vi "THzTimeScan_830.vi"(0 "input":T1) -> (1 "loop stop":bool, 2 "x-axis":sgl[](array[numeric]), 3 "y-axis":dbl[](array[numeric]))   [LabVIEW 2010]
panel:
  out "Array":dbl[](array[numeric])
  out "String":string
  out "Read position":bool
  out "Ask position":bool
  out "Move delay":bool
  out "Read830":bool
  out "Command":string
  out "THz Signal Graph":dbl(graph)
  in  "loop stop":bool
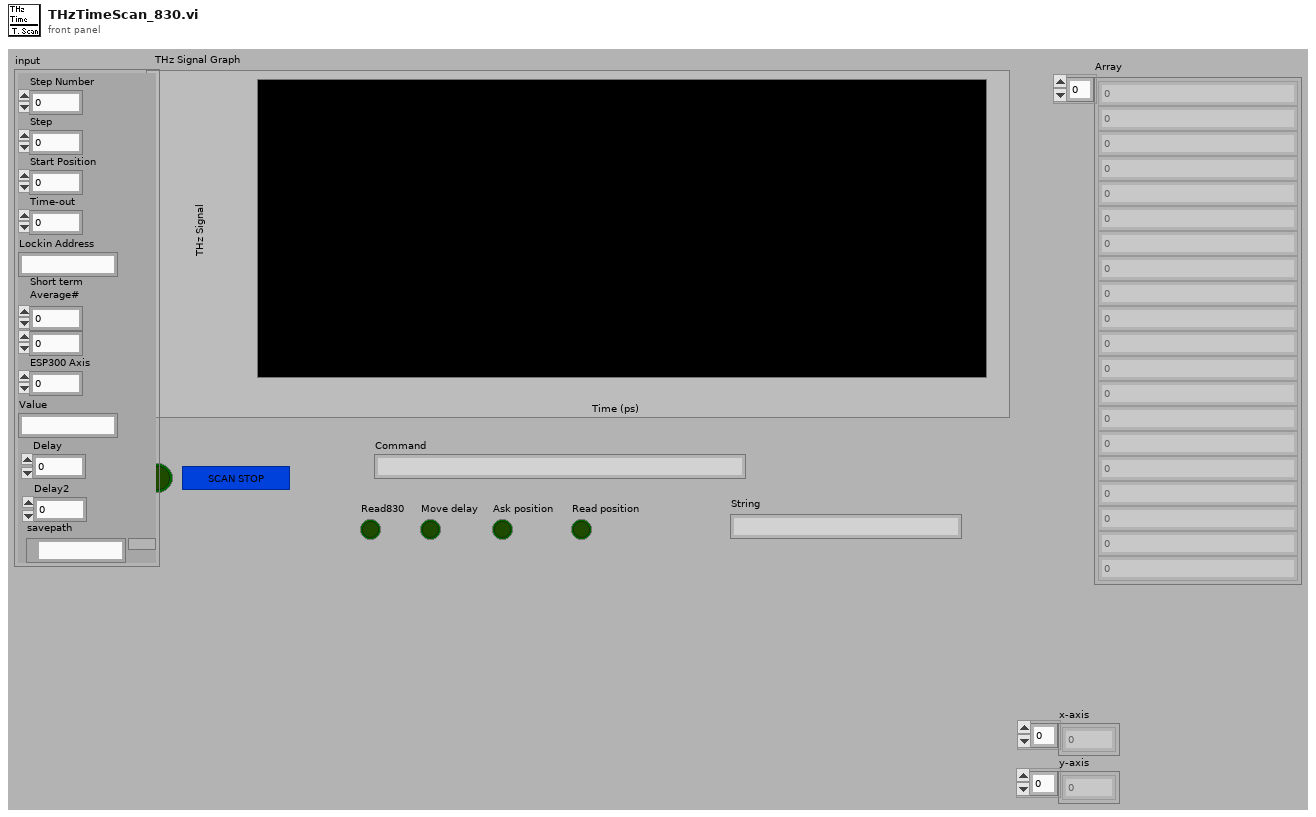
[diagram p1: front panel]
types:
  T1 = cluster{"Step Number":i32, "Step":sgl, "Start Position":sgl, "Time-out":i32, "Lockin Address":string, "Short term \nAverage#":i8, i32, "ESP300 Axis":i8, "Value":string, "Delay":dbl, "Delay2":dbl, "savepath":path}
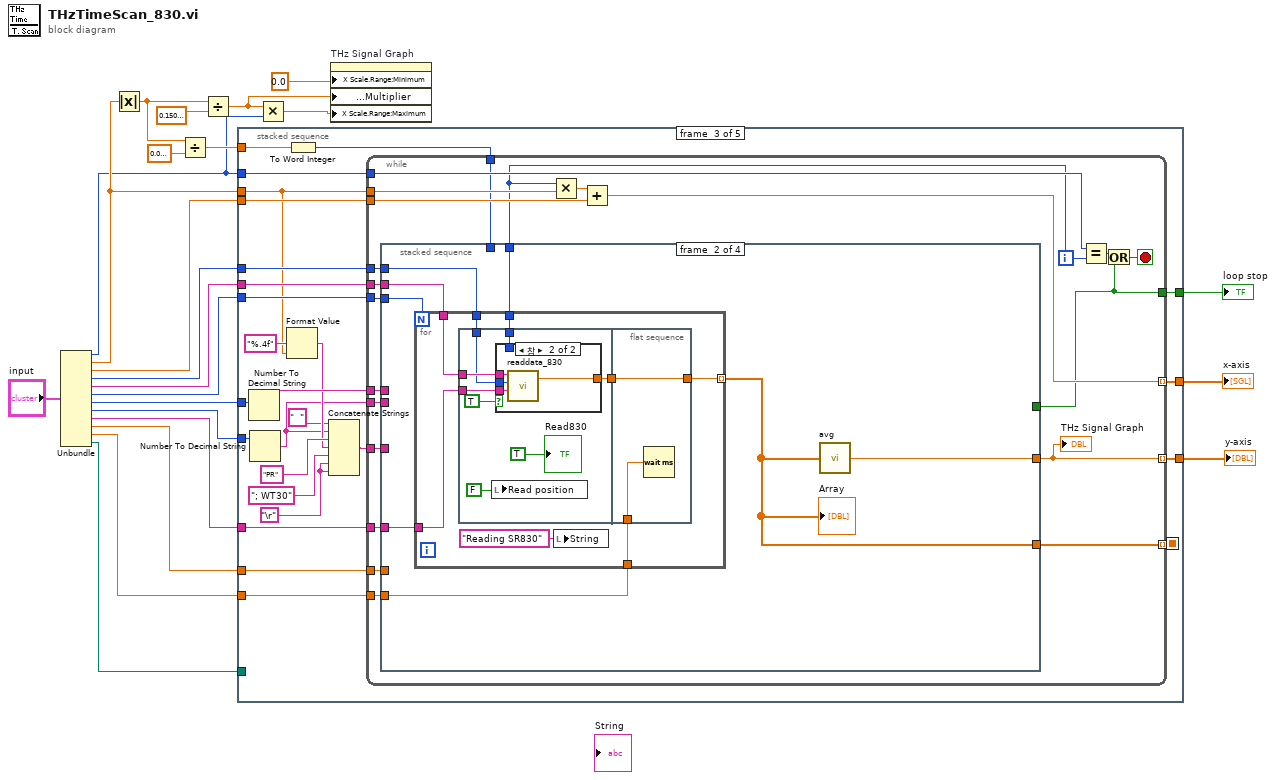
[diagram p0: block diagram]
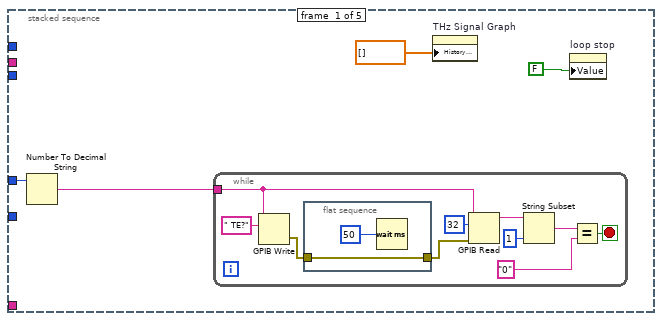
[diagram p2: hidden frame]
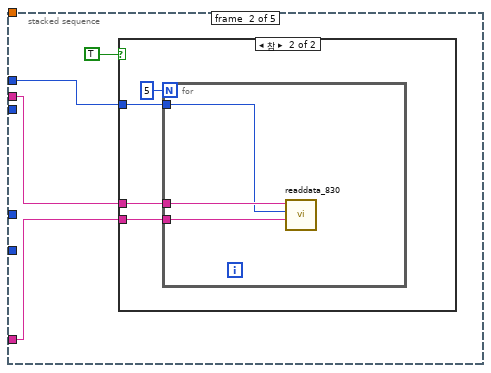
[diagram p3: hidden frame]
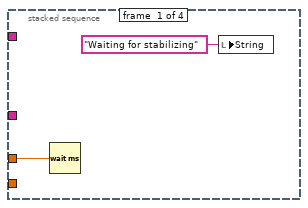
[diagram p5: hidden frame]
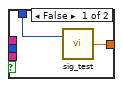
[diagram p6: hidden frame]
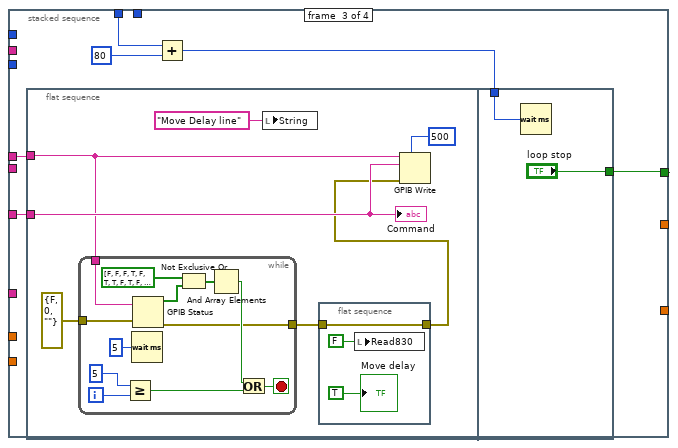
[diagram p7: hidden frame]
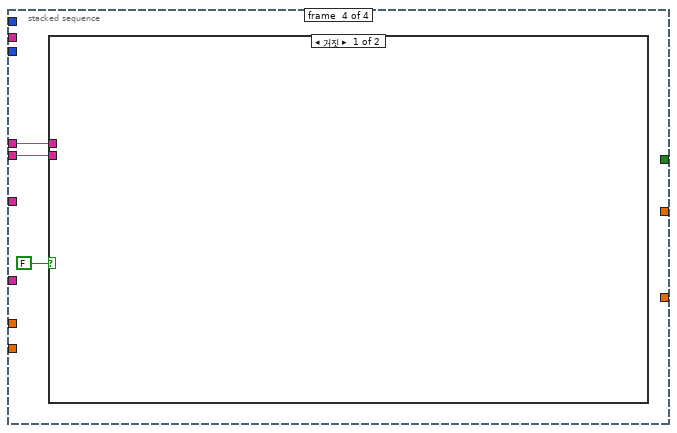
[diagram p8: hidden frame]
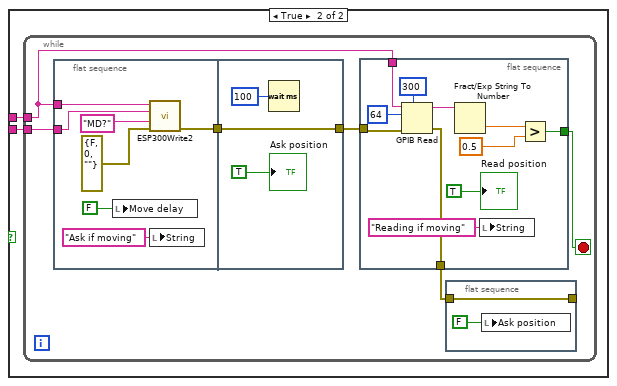
[diagram p9: hidden frame]
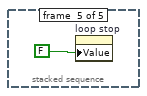
[diagram p11: hidden frame]
diagram:
  n1 = Unbundle("input") -> ("Step Number"=w8:i32, "Step"=w15:sgl, "Start Position"=w14:sgl, "Time-out"=w13:i32, "Lockin Address"=w12:string, "Short term \nAverage#"=w4:i8, w11:i32, "ESP300 Axis"=w10:i8, "Value"=w9:string, "Delay"=w3:dbl, "Delay2"=w2:dbl, "savepath"=w1:path)
  n2 = Absolute Value(x=w15) -> (abs(x)=w19:sgl)
  n3 = Divide(x=w19, y=sgl 0.004) -> (x/y=w17:sgl)
  n4 = Divide(x=w19, y=sgl 0.15) -> (x/y=w6:sgl)
  n5 = stacked-sequence {
    seq-local: [_ _ w52 _ _] -> [_ _ _ _ _]
    tunnel: w14 -> [_ _ w76 _ _]
    tunnel: w13 -> [_ w43 w75 _ _]
    tunnel: w12 -> [_ w42 w74 _ _]
    tunnel: w4 -> [_ _ w73 _ _]
    tunnel: w11 -> [w25 _ w68 _ _]
    tunnel: w10 -> [_ _ w66 _ _]
    tunnel: w9 -> [_ w41 w58 _ _]
    tunnel: [_ _ w72 _ _] -> w23
    tunnel: [_ _ w71 _ _] -> w22
    tunnel: [_ _ w70 _ _] -> w21
    tunnel: w15 -> [_ _ w64 _ _]
    tunnel: w8 -> [_ _ w69 _ _]
    tunnel: w17 -> [_ _ w63 _ _]
    tunnel: w3 -> [_ _ w54 _ _]
    tunnel: w2 -> [_ _ w53 _ _]
    tunnel: w1 -> [_ _ _ _ _]
    frame #0 {
      n6 = Number To Decimal String(number=w25) -> (decimal integer string=w24:string)  [unwired: 1 in]
      n7 = while {
        tunnel: w24 -> [w30]
        stop <- w35 stop-if-true
        n8 = GPIB Write(0:w30, 1:" TE?" ("data")) -> (6:w29:errorcluster)  [unwired: 3 in, 1 out]
        n9 = flat-sequence {
          tunnel: w29 -> [w39]
          tunnel: [w39] -> w28
          frame #0 {
            n10 = Wait (ms)(milliseconds to wait=u32 50) -> ()  [unwired: 1 out]
          }
        }
        n11 = GPIB Read(0:w30, 1:32 ("byte count"), 3:w28) -> (5:w34:string)  [unwired: 2 in, 2 out]
        n12 = String Subset(string=w34, length (rest)=1 ("offset (0)")) -> (substring=w32:string)  [unwired: 1 in]
        n13 = Equal?(x=w32, y="0") -> (x = y?=w35:bool)
      }
      n14 = property on="THz Signal Graph" class="WFChart (엄격한)"("History Data"=dbl[] []) -> ()  [unwired: 2 in, 2 out]
      n15 = property on="loop stop" class="Bool (엄격한)"("Value"=FALSE) -> ()  [unwired: 2 in, 2 out]
    }
    frame #1 {
      n16 = case shown="참" TRUE {
        tunnel: w43 -> [_ w46]
        tunnel: w42 -> [_ w45]
        tunnel: w41 -> [_ w44]
        frame False {
        }
        frame True {
          n17 = for {
            N: 5 -> [_]
            tunnel: w45 -> [w50]
            tunnel: w44 -> [w49]
            tunnel: w46 -> [w48]
            n18 = call "readdata_830.vi"("Command"=w49, "timeout"=w48, "Lockin Address"=w50) -> ()  [unwired: 1 in, 2 out]
          }
        }
      }
    }
    frame #2 {
      w57 = "\r"
      n19 = Number To Decimal String(number=w68) -> (decimal integer string=w67:string)  [unwired: 1 in]
      n20 = Number To Decimal String(number=w66) -> (decimal integer string=w55:string)  [unwired: 1 in]
      n21 = Format Value(format string="%.4f", value (0)=w64) -> (output string=w60:string)  [unwired: 1 in]
      n22 = To Word Integer(number=w63) -> (16bit integer=w62:i16)
      n23 = Concatenate Strings("  " ("string"), w55, "PR" ("Substring"), w60, "; WT30" ("string"), w57, w57) -> (w51:string)
      n24 = while {
        tunnel: [w82] -> w72
        tunnel: [w88] -> w70 mode=indexing
        tunnel: [w94] -> w71 mode=indexing
        tunnel: w69 -> [w93]
        tunnel: w64 -> [w92]
        tunnel: w76 -> [w91]
        tunnel: w75 -> [w83]
        tunnel: w74 -> [w90]
        tunnel: w73 -> [w89]
        tunnel: w67 -> [w87]
        tunnel: w51 -> [w86]
        tunnel: w62 -> [w85]
        tunnel: w58 -> [w84]
        tunnel: w55 -> [w81]
        tunnel: w54 -> [w80]
        tunnel: w53 -> [w79]
        tunnel: [w78] -> w52 mode=indexing
        i -> [w77]
        stop <- w97 stop-if-true
        n25 = stacked-sequence {
          tunnel: w90 -> [_ w104 _ _]
          tunnel: [_ w106 _ _] -> w88
          tunnel: w89 -> [_ w107 _ _]
          tunnel: w87 -> [_ _ w136 w164]
          tunnel: w86 -> [_ _ w137 _]
          tunnel: w85 -> [_ _ w135 _]
          tunnel: w84 -> [_ w105 _ _]
          tunnel: w83 -> [_ w103 _ _]
          tunnel: [_ _ w132 _] -> w82
          tunnel: w81 -> [_ _ _ w163]
          tunnel: w80 -> [w99 _ _ _]
          tunnel: w79 -> [_ w102 _ _]
          tunnel: [_ w101 _ _] -> w78
          tunnel: w77 -> [_ w100 _ _]
          frame #0 {
            n26 = Wait (ms)(milliseconds to wait=w99) -> ()  [unwired: 1 out]
            n27 = local write "String"("Waiting for stabilizing" ("String")) -> ()
          }
          frame #1 {
            n28 = for {
              N: w107 -> [_]
              tunnel: w104 -> [w112]
              tunnel: w103 -> [w115]
              tunnel: [w114] -> w101 mode=indexing
              tunnel: w105 -> [w113]
              tunnel: w102 -> [w109]
              tunnel: w100 -> [w108]
              n29 = flat-sequence {
                tunnel: w115 -> [w119]
                tunnel: w113 -> [w120]
                tunnel: w112 -> [w121]
                tunnel: [w118] -> w110
                tunnel: w108 -> [w116]
                tunnel: [w131] -> w114
                tunnel: w110 -> [w131]
                tunnel: w109 -> [w130]
                frame #0 {
                  n30 = local write "Read position"(FALSE ("Read position")) -> ()
                  n31 = case shown="참" TRUE {
                    tunnel: w121 -> [_ w129]
                    tunnel: w120 -> [_ w128]
                    tunnel: w119 -> [_ w127]
                    tunnel: [w125 w126] -> w118
                    tunnel: w116 -> [w124 _]
                    frame False {
                      n32 = call "sig_test.vi"("index (row)"=w124) -> ("element"=w125:dbl)  [unwired: 1 in]
                    }
                    frame True {
                      n33 = call "readdata_830.vi"("Command"=w128, "timeout"=w127, "Lockin Address"=w129) -> ("Data"=w126:dbl)  [unwired: 1 in, 1 out]
                    }
                  }
                  "Read830" <- TRUE ("Read830")
                }
                frame #1 {
                  n34 = Wait (ms)(milliseconds to wait=w130) -> ()  [unwired: 1 out]
                }
              }
              n35 = local write "String"("Reading SR830" ("String")) -> ()
            }
            "Array" <- w101
            n36 = call "avg.vi"("Array"=w101) -> ("Numeric"=w106:dbl)
          }
          frame #2 {
            n37 = flat-sequence {
              tunnel: w137 -> [w144]
              tunnel: w136 -> [w142]
              tunnel: w134 -> [w160]
              tunnel: ["loop stop"] -> w132
              frame #0 {
                n38 = while {
                  tunnel: errorcluster {"status"=FALSE, "code"=0, "source"=""} ("error in (no error)") -> [w159]
                  tunnel: [w149] -> w139
                  tunnel: w142 -> [w148]
                  i -> [w158]
                  stop <- w155 stop-if-true
                  n39 = Greater Or Equal?(x=5, y=w158) -> (x >= y?=w156:bool)
                  n40 = Wait (ms)(milliseconds to wait=u32 5) -> ()  [unwired: 1 out]
                  n41 = GPIB Status(0:w148, 1:w159) -> (2:w153:bool[], 5:w149:errorcluster)  [unwired: 2 out]
                  n42 = Not Exclusive Or(1:w153, 2:bool[] [FALSE, FALSE, FALSE, TRUE, FALSE, TRUE, TRUE, FALSE, TRUE, FALSE, FALSE, FALSE, FALSE, FALSE, FALSE, FALSE] ("status 2")) -> (0:w152:bool[])
                  n43 = And Array Elements(Boolean array=w152) -> (logical AND=w151:bool)
                  n44 = Or(x=w151, y=w156) -> (x .or. y?=w155:bool)
                }
                n45 = local write "String"("Move Delay line" ("String")) -> ()
                n46 = flat-sequence {
                  tunnel: [w147] -> w140
                  tunnel: w139 -> [w147]
                  frame #0 {
                    n47 = local write "Read830"(FALSE ("Read830")) -> ()
                    "Move delay" <- TRUE ("Move delay")
                  }
                }
                n48 = GPIB Write(0:w142, 1:w144, 3:w140, 4:500 ("timeout ms (488.2 global)")) -> ()  [unwired: 1 in, 2 out]
                "Command" <- w144
              }
              frame #1 {
                n49 = Wait (ms)(milliseconds to wait=w160) -> ()  [unwired: 1 out]
              }
            }
            n50 = Add(x=w135, y=i16 80) -> (x+y=w134:i16)
          }
          frame #3 {
            n51 = case shown="거짓" FALSE {
              tunnel: w164 -> [_ w166]
              tunnel: w163 -> [_ w165]
              frame False {
              }
              frame True {
                n52 = while {
                  tunnel: w166 -> [w168]
                  tunnel: w165 -> [w172]
                  stop <- w170 stop-if-true
                  n53 = flat-sequence {
                    tunnel: w172 -> [w186]
                    tunnel: w168 -> [w189]
                    tunnel: [w190] -> w169
                    tunnel: [w195] -> w171
                    tunnel: w169 -> [w195]
                    frame #0 {
                      n54 = local write "Move delay"(FALSE ("Move delay")) -> ()
                      n55 = call "ESP300Write2.vi"("error in (no error)"=errorcluster {"status"=FALSE, "code"=0, "source"=""}, "Command"="MD?", "ESP300 Channel"=w186, "ESP300 Address"=w189) -> ("error out"=w190:errorcluster)  [unwired: 3 in]
                      n56 = local write "String"("Ask if moving" ("String")) -> ()
                    }
                    frame #1 {
                      n57 = Wait (ms)(milliseconds to wait=u32 100) -> ()  [unwired: 1 out]
                      "Ask position" <- TRUE ("Ask position")
                    }
                  }
                  n58 = flat-sequence {
                    tunnel: w171 -> [w185]
                    tunnel: [w182] -> w170
                    tunnel: w168 -> [w178]
                    tunnel: [w176] -> w167
                    frame #0 {
                      n59 = GPIB Read(0:w178, 1:64 ("byte count"), 3:w185, 4:300 ("timeout ms (488.2 global)")) -> (5:w181:string, 7:w176:errorcluster)  [unwired: 1 in, 1 out]
                      n60 = Fract/Exp String To Number(string=w181) -> (number=w180:dbl)  [unwired: 3 in, 1 out]
                      n61 = local write "String"("Reading if moving" ("String")) -> ()
                      n62 = Greater?(x=w180, y=0.5) -> (0:w182:bool)
                      "Read position" <- TRUE ("Read position")
                    }
                  }
                  n63 = flat-sequence {
                    tunnel: [w174] -> _
                    tunnel: w167 -> [w174]
                    frame #0 {
                      n64 = local write "Ask position"(FALSE ("Ask position")) -> ()
                    }
                  }
                }
              }
            }
          }
        }
        "THz Signal Graph" <- w88
        n65 = Multiply(x=w77, y=w92) -> (x*y=w95:sgl)
        n66 = Add(x=w95, y=w91) -> (x+y=w94:sgl)
        n67 = Equal?(x=w93, y=w77) -> (x = y?=w96:bool)
        n68 = Or(x=w96, y=w82) -> (x .or. y?=w97:bool)
      }
    }
    frame #3 {
    }
    frame #4 {
      n69 = property on="loop stop" class="Bool (엄격한)"("Value"=FALSE) -> ()  [unwired: 2 in, 2 out]
    }
  }
  "loop stop" <- w23
  "x-axis" <- w22
  "y-axis" <- w21
  n70 = Multiply(x=w6, y=w8) -> (x*y=w5:sgl)
  n71 = property on="THz Signal Graph" class="WFChart (엄격한)"("X Scale.Range:Minimum"=0.0, "X Scale.Offset and Multiplier:Multiplier"=w6, "X Scale.Range:Maximum"=w5) -> ()  [unwired: 2 in, 2 out]
